vi "Add State to Routing Channel.vi"(8 "error in (no error)":errorcluster, 10 "Routing State":T1, 11 "Channel Ref in":T3 format="%.0x") -> (0 "error out":errorcluster, 3 "Channel Ref out":T3=18446744073709551615 format="%.0x")   [LabVIEW 2017, in "SLSC Switch Scripting.lvlib"]
uses:
  SLSC Switch Scripting.lvlib
  <vilib>/NI Veristand/Custom Device API/Custom Device Item Ref.ctl
  Routing State.ctl
  Connection.ctl
  <vilib>/NI VeriStand/Custom Device API/Custom Device API.lvlib
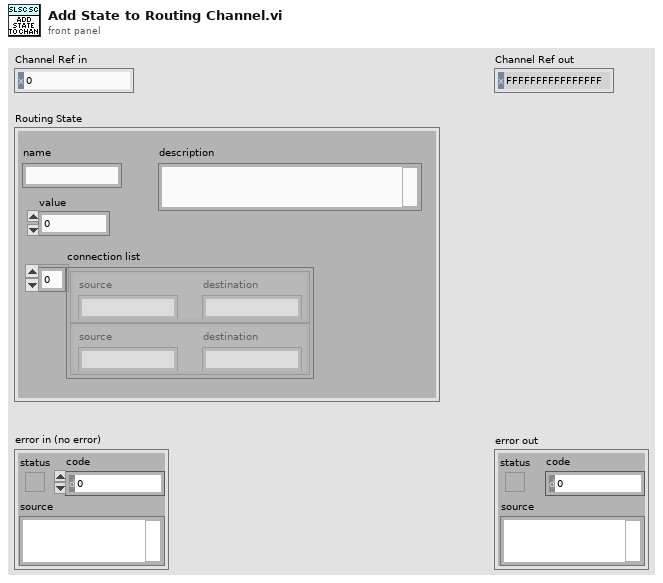
[diagram p1: front panel]
types:
  T1 = typedef "SLSC Switch Scripting.lvlib/Routing State.ctl" = cluster{"name":string, "description":string, "value":i32, "connection list":T2[]}
  T2 = typedef "SLSC Switch Scripting.lvlib/Connection.ctl" = cluster{"source":string, "destination":string}
  T3 = typedef "Custom Device API.lvlib/Custom Device Item Ref.ctl" = u64
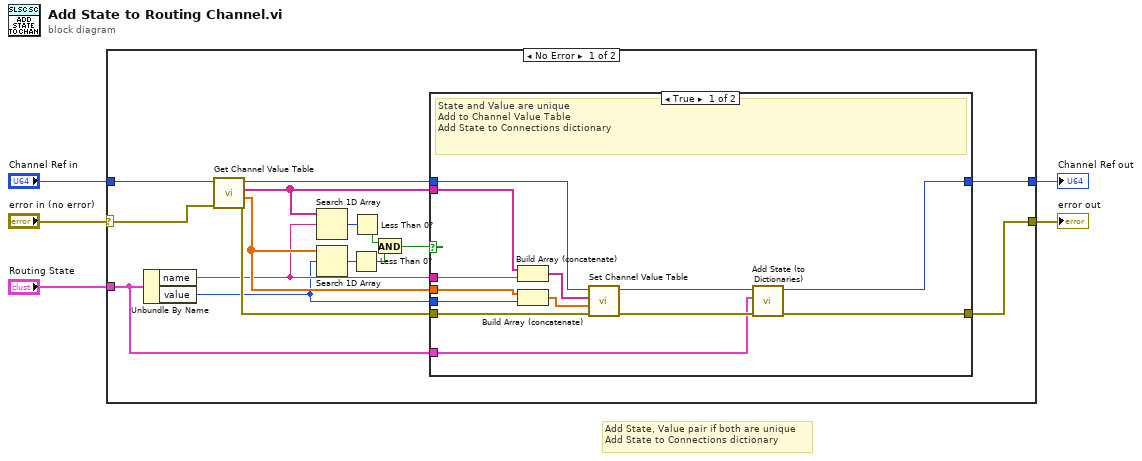
[diagram p0: block diagram]
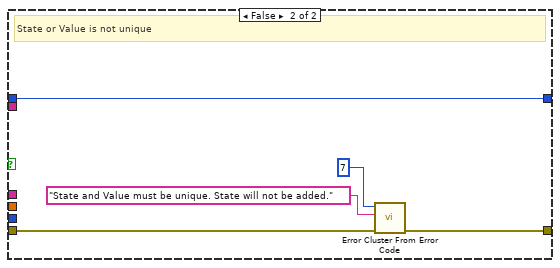
[diagram p2: hidden frame]
diagram:
  # "Add State, Value pair if both are unique\nAdd State to Connections dictionary"
  n1 = case shown="No Error" "error in (no error)" {
    selector: "error in (no error)" -> [w20 w41]
    tunnel: [w16 w41] -> w2
    tunnel: "Channel Ref in" -> [w21 w40]
    tunnel: [w17 w40] -> w3
    tunnel: "Routing State" -> [w6 _]
    frame No Error {
      n2 = Unbundle By Name(w6) -> ("name"=w8:string, "value"=w7:i32)
      n3 = call "Get Channel Value Table.vi"("error in (no error)"=w20, "Channel Ref in"=w21) -> ("error out"=w18:errorcluster, "Values"=w14:dbl[], "States"=w15:string[], "Channel Ref out"=w19:T3)  [unwired: 6 in]
      n4 = Search 1D Array(1D array=w15, element=w8) -> (index of element=w13:i32)  [unwired: 1 in]
      n5 = Search 1D Array(1D array=w14, element=w7) -> (index of element=w12:i32)  [unwired: 1 in]
      n6 = Less Than 0?(x=w12) -> (x < 0?=w10:bool)
      n7 = Less Than 0?(x=w13) -> (x < 0?=w11:bool)
      n8 = And(x=w11, y=w10) -> (x .and. y?=w9:bool)
      n9 = case shown="True" w9 {
        tunnel: w19 -> [w31 w35]
        tunnel: w18 -> [w30 w37]
        tunnel: w14 -> [w33 _]
        tunnel: [w26 w35] -> w17
        tunnel: [w23 w36] -> w16
        tunnel: w7 -> [w34 _]
        tunnel: w15 -> [w32 _]
        tunnel: w8 -> [w25 _]
        tunnel: w6 -> [w22 _]
        frame True {
          # "State and Value are unique\nAdd to Channel Value Table\nAdd State to Connections dictionary"
          n10 = Build Array (concatenate)(w32, w25) -> (w29:string[])
          n11 = Build Array (concatenate)(w33, w34) -> (w28:dbl[])
          n12 = call "Set Channel Value Table.vi"("error in (no error)"=w30, "Values"=w28, "States"=w29, "Channel Ref in"=w31) -> ("error out"=w24:errorcluster, "Channel Ref out"=w27:T3)  [unwired: 6 in]
          n13 = call "Add State (to Dictionaries).vi"("error in (no error)"=w24, "Routing State"=w22, "Channel Ref in"=w27) -> ("error out"=w23:errorcluster, "Channel Ref out"=w26:T3)  [unwired: 7 in]
        }
        frame False {
          # "State or Value is not unique"
          n14 = call <vilib>:"Error Cluster From Error Code.vi"("error in (no error)"=w37, "error message (\"\")"="State and Value must be unique. State will not be added." ("error message (\"\")"), "error code (0)"=7) -> ("error out"=w36:errorcluster)  [unwired: 6 in]
        }
      }
    }
    frame Error {
    }
  }
  "Channel Ref out" <- w3
  "error out" <- w2
